vi "MTS_ClearWSTree.vi"(8 "error in":errorcluster, 11 "Tree Refnum":refnum<vi>) -> (0 "error out":errorcluster, 3 "Tree Refnum (dup)":refnum<vi>)   [LabVIEW 8.6]
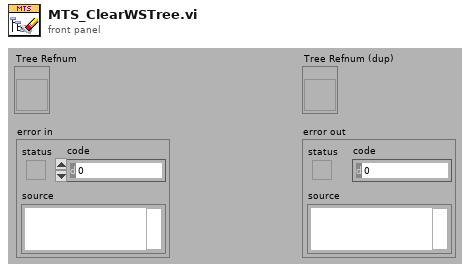
[diagram p1: front panel]
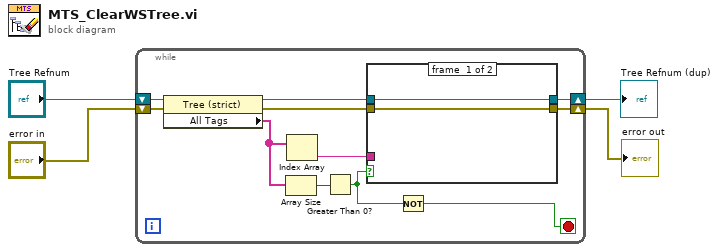
[diagram p0: block diagram]
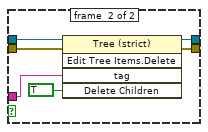
[diagram p2: hidden frame]
diagram:
  n1 = while {
    shift-right: [w12] -> w3
    shift-left: "error in" -> [w9]
    shift-right: [w11] -> w4
    shift-left: "Tree Refnum" -> [w10]
    stop <- w5 stop-if-true
    n2 = property on="Property Node" class="Tree (strict)"(reference=w10, error in=w9) -> (reference out=w14:refnum<vi>, error out=w13:errorcluster, "All Tags"=w8:string[])
    n3 = Array Size(array=w8) -> (size(s)=w7:i32)
    n4 = Index Array(array=w8) -> (element=w15:string)  [unwired: 1 in]
    n5 = Greater Than 0?(x=w7) -> (x > 0?=w6:bool)
    n6 = case shown="True" w6 {
      tunnel: w15 -> [_ w23]
      tunnel: w14 -> [w16 w22]
      tunnel: w13 -> [w17 w21]
      tunnel: [w17 w19] -> w12
      tunnel: [w16 w18] -> w11
      frame #0 {
      }
      frame #1 {
        n7 = invoke on="Invoke Node" class="Tree (strict)" method="Edit Tree Items.Delete"(reference=w22, error in=w21, "tag"=w23, "Delete Children"=TRUE ("Delete Children?")) -> (reference out=w18:refnum<vi>, error out=w19:errorcluster)  [unwired: 1 in, 3 out]
      }
    }
    n8 = Not(x=w6) -> (.not. x?=w5:bool)
  }
  "Tree Refnum (dup)" <- w4
  "error out" <- w3
